vi "test_UART_1.vi"() -> ()   [LabVIEW 2014]
uses:
  <vilib>/myRIO/Instrument Drivers/Onboard IO/UART/typedef/VISA Configuration.ctl
  <vilib>/Instr/_visa.llb/VISA Configure Serial Port (Instr).vi
  <vilib>/myRIO/Instrument Drivers/Onboard IO/UART/UART.lvlib
panel:
  out "error out 2":errorcluster
  out "Characters Read":string
  in  "error in (no error)":errorcluster
  out "Character Count":u32
  in  "Characters to Write":string
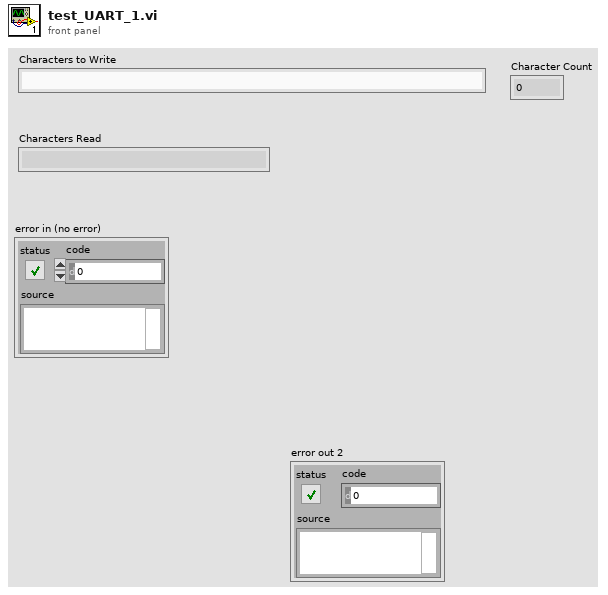
[diagram p1: front panel]
types:
  T1 = typedef "UART.lvlib/VISA Configuration.ctl" = cluster{"baud rate (9600)":u32, "data bits (8)":u16, "parity (0:none)":enum16{"None", "Odd", "Even", "Mark", "Space"}, "stop bits (10: 1 bit)":u16, "flow control (0:none)":u16, "termination char\n(0xA = '\\n' = LF) ":u8, "Enable Termination\nChar (T)":bool, "timeout (10sec)":u32}
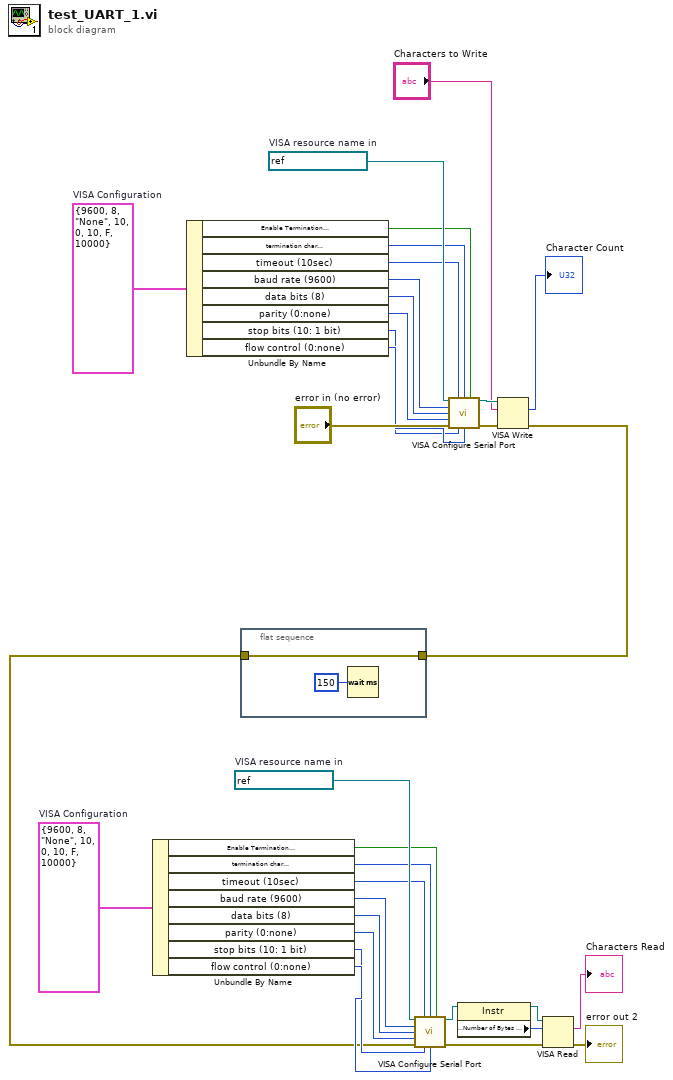
[diagram p0: block diagram]
diagram:
  w17 = T1 {"baud rate (9600)"=9600, "data bits (8)"=8, "parity (0:none)"=enum."None", "stop bits (10: 1 bit)"=10, "flow control (0:none)"=0, "termination char\n(0xA = '\\n' = LF) "=10, "Enable Termination\nChar (T)"=FALSE, "timeout (10sec)"=10000}  # VISA Configuration
  w18 = refnum<visa-resource-name> "ASRL1::INSTR"  # VISA resource name in
  w32 = T1 {"baud rate (9600)"=9600, "data bits (8)"=8, "parity (0:none)"=enum."None", "stop bits (10: 1 bit)"=10, "flow control (0:none)"=0, "termination char\n(0xA = '\\n' = LF) "=10, "Enable Termination\nChar (T)"=FALSE, "timeout (10sec)"=10000}  # VISA Configuration
  w33 = refnum<visa-resource-name> "ASRL2::INSTR"  # VISA resource name in
  n1 = Unbundle By Name(w17) -> ("Enable Termination\nChar (T)"=w12:bool, "termination char\n(0xA = '\\n' = LF)"=w11:u8, "timeout (10sec)"=w10:u32, "baud rate (9600)"=w5:u32, "data bits (8)"=w6:u16, "parity (0:none)"=w7:enum16{"None", "Odd", "Even", "Mark", "Space"}, "stop bits (10: 1 bit)"=w8:u16, "flow control (0:none)"=w9:u16)
  n2 = Unbundle By Name(w32) -> ("Enable Termination\nChar (T)"=w28:bool, "termination char\n(0xA = '\\n' = LF)"=w27:u8, "timeout (10sec)"=w26:u32, "baud rate (9600)"=w21:u32, "data bits (8)"=w22:u16, "parity (0:none)"=w23:enum16{"None", "Odd", "Even", "Mark", "Space"}, "stop bits (10: 1 bit)"=w24:u16, "flow control (0:none)"=w25:u16)
  n3 = flat-sequence {
    tunnel: w2 -> [w34]
    tunnel: [w34] -> w1
    frame #0 {
      n4 = Wait (ms)(milliseconds to wait=u32 150) -> ()  [unwired: 1 out]
    }
  }
  n5 = call-poly "VISA Configure Serial Port"("VISA resource name"=w18, "timeout (10sec)"=w10, "termination char\n(0xA = '\\n' = LF)"=w11, "Enable Termination\nChar (T)"=w12, "baud rate (9600)"=w5, "data bits (8)"=w6, "parity (0:none)"=w7, "error in (no error)"=w1, "stop bits (10: 1 bit)"=w8, "flow control (0:none)"=w9) -> ("VISA resource name out"=w15:refnum<visa-resource-name>, "error out"=w14:errorcluster)  [unwired: 4 in]
  n6 = call-poly "VISA Configure Serial Port"("VISA resource name"=w33, "timeout (10sec)"=w26, "termination char\n(0xA = '\\n' = LF)"=w27, "Enable Termination\nChar (T)"=w28, "baud rate (9600)"=w21, "data bits (8)"=w22, "parity (0:none)"=w23, "error in (no error)"="error in (no error)", "stop bits (10: 1 bit)"=w24, "flow control (0:none)"=w25) -> ("VISA resource name out"=w30:refnum<visa-resource-name>, "error out"=w29:errorcluster)  [unwired: 4 in]
  n7 = property class="Instr"(reference=w15) -> (reference out=w3:refnum<visa-resource-name>, "Serial Settings:Number of Bytes at Serial Port"=w4:u32)  [unwired: 1 in, 1 out]
  n8 = VISA Write(VISA resource name=w30, write buffer="Characters to Write", error in (no error)=w29) -> (return count=→"Character Count":u32, error out=w2:errorcluster)  [unwired: 1 out]
  n9 = VISA Read(VISA resource name=w3, byte count=w4, error in (no error)=w14) -> (read buffer=→"Characters Read":string, error out=→"error out 2":errorcluster)  [unwired: 2 out]
